vi "SetPara_BP4610.vi"(8 "error in":errorcluster, 10 "SetBP":T1={"Set"=enum."FREQ/WAVE", "Operation mode"=0, "Voltage[Vp-p]"=0.0, "Current[Ap-p]"=0.0, "Voltage[V]"=0.0, "Current[A]"=0.0, "Frequency[Hz]"=1.0, "Waveform"=enum."Sine"} {"Frequency[Hz]" min=1.0 max=100000.0 step=0.1; "Current[A]" min=-20.0 max=20.0 step=0.001; "Voltage[V]" min=-115.0 max=115.0 step=0.01; "Current[Ap-p]" min=0.0 max=60.0 step=0.01; "Voltage[Vp-p]" min=0.0 max=120.0 step=0.1; "Operation mode" items=["CV-INT", "CV-EXT", "CV-ADD", "CC-INT", "CC-EXT", "CC-ADD"]}, 11 "VISA":refnum<visa-resource-name> caption="VISAsession") -> (0 "error out":errorcluster, 3 "VISA out":refnum<visa-resource-name>)   [LabVIEW 2019]
uses:
  Type def/SetNF_BP4610.ctl
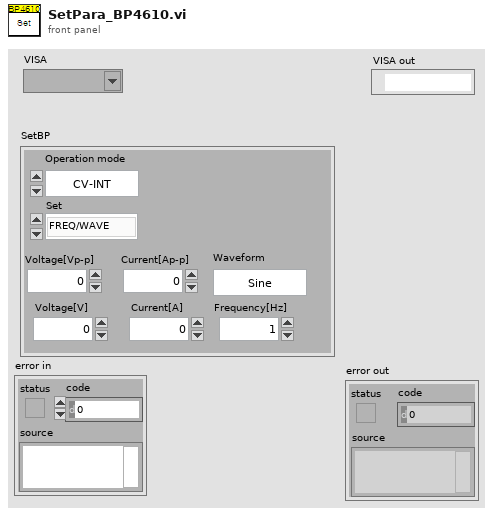
[diagram p1: front panel]
types:
  T1 = typedef "SetNF_BP4610.ctl" = cluster{"Set":enum16{"Current", "Voltage", "FREQ/WAVE"}, "Operation mode":u16, "Voltage[Vp-p]":dbl, "Current[Ap-p]":dbl, "Voltage[V]":dbl, "Current[A]":dbl, "Frequency[Hz]":dbl, "Waveform":enum16{"Sine", "Square", "ARB 1", "ARB 2", "ARB 3", "ARB 4", "ARB 5", "ARB 6", "ARB 7", "ARB 8", "ARB 9", "ARB 10", "ARB 11", "ARB 12", "ARB 13", "ARB 14", "ARB 15", "ARB 16"}}
  T2 = enum16{"Sine", "Square", "ARB 1", "ARB 2", "ARB 3", "ARB 4", "ARB 5", "ARB 6", "ARB 7", "ARB 8", "ARB 9", "ARB 10", "ARB 11", "ARB 12", "ARB 13", "ARB 14", "ARB 15", "ARB 16"}
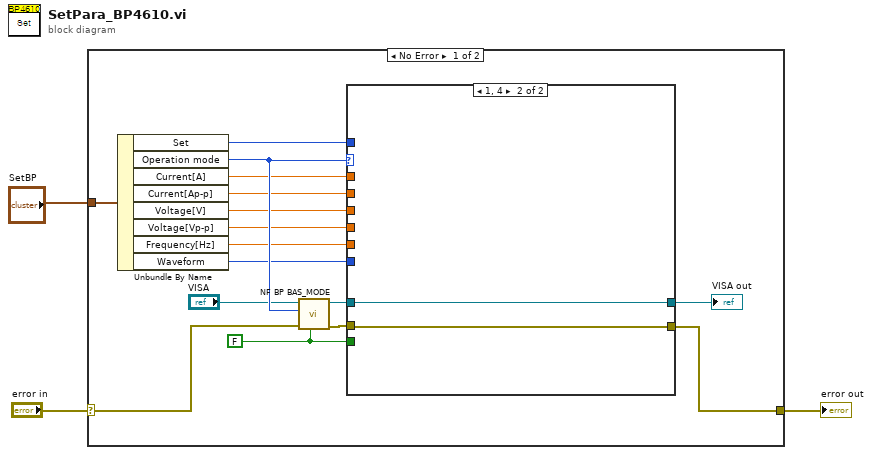
[diagram p0: block diagram]
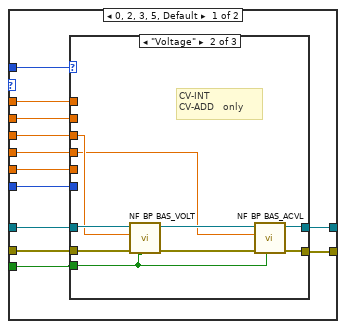
[diagram p2: hidden frame]
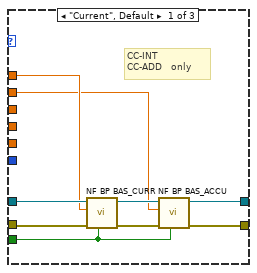
[diagram p3: hidden frame]
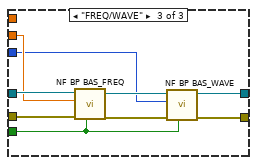
[diagram p4: hidden frame]
diagram:
  n1 = case shown="No Error" "error in" {
    selector: "error in" -> [w11 w61]
    tunnel: [w10 w61] -> w2
    tunnel: "SetBP" -> [w16 _]
    frame No Error {
      w17 = FALSE ("Read")
      n2 = Unbundle By Name(w16) -> ("Set"=w14:enum16{"Current", "Voltage", "FREQ/WAVE"}, "Operation mode"=w15:u16, "Current[A]"=w13:dbl, "Current[Ap-p]"=w12:dbl, "Voltage[V]"=w9:dbl, "Voltage[Vp-p]"=w8:dbl, "Frequency[Hz]"=w7:dbl, "Waveform"=w6:T2)
      n3 = call <instrlib>:"NF BP BAS_MODE.vi"("Read(F)"=w17, "error in (no error)"=w11, "Select Mode"=w15, "VISAsession"="VISA") -> ("error out"=w18:errorcluster, "CopyVISAsession"=w19:refnum<visa-resource-name>)  [unwired: 4 in, 2 out]
      n4 = case shown="1, 4" w15 {
        tunnel: w19 -> [w31 w60]
        tunnel: w18 -> [w30 w59]
        tunnel: [w29 w60] -> w4
        tunnel: [w28 w59] -> w10
        tunnel: w17 -> [w27 _]
        tunnel: w14 -> [w26 _]
        tunnel: w13 -> [w25 _]
        tunnel: w12 -> [w24 _]
        tunnel: w9 -> [w23 _]
        tunnel: w8 -> [w22 _]
        tunnel: w7 -> [w21 _]
        tunnel: w6 -> [w20 _]
        frame 0, 2, 3, 5, Default {
          n5 = case shown="\"Voltage\"" w26 {
            tunnel: w30 -> [w38 w49 w58]
            tunnel: w31 -> [w36 w45 w54]
            tunnel: [w40 w47 w55] -> w28
            tunnel: w27 -> [w37 w46 w56]
            tunnel: [w34 w43 w52] -> w29
            tunnel: w25 -> [w33 _ _]
            tunnel: w24 -> [w32 _ _]
            tunnel: w23 -> [_ w42 _]
            tunnel: w22 -> [_ w41 _]
            tunnel: w21 -> [_ _ w51]
            tunnel: w20 -> [_ _ w50]
            frame "Current", Default {
              # "CC-INT\nCC-ADD   only"
              n6 = call <instrlib>:"NF BP BAS_CURR.vi"("Read(F)"=w37, "error in (no error)"=w38, "Current[A]"=w33, "VISAsession"=w36) -> ("error out"=w39:errorcluster, "CopyVISAsession"=w35:refnum<visa-resource-name>)  [unwired: 4 in, 2 out]
              n7 = call <instrlib>:"NF BP BAS_ACCU.vi"("Read(F)"=w37, "error in (no error)"=w39, "Current[Ap-p]"=w32, "VISAsession"=w35) -> ("error out"=w40:errorcluster, "CopyVISAsession"=w34:refnum<visa-resource-name>)  [unwired: 4 in, 2 out]
            }
            frame "Voltage" {
              # "CV-INT\nCV-ADD   only"
              n8 = call <instrlib>:"NF BP BAS_VOLT.vi"("Read(F)"=w46, "error in (no error)"=w49, "Voltage[V]"=w42, "VISAsession"=w45) -> ("error out"=w48:errorcluster, "CopyVISAsession"=w44:refnum<visa-resource-name>)  [unwired: 4 in, 2 out]
              n9 = call <instrlib>:"NF BP BAS_ACVL.vi"("Read(F)"=w46, "error in (no error)"=w48, "Voltage[Vp-p]"=w41, "VISAsession"=w44) -> ("error out"=w47:errorcluster, "CopyVISAsession"=w43:refnum<visa-resource-name>)  [unwired: 4 in, 2 out]
            }
            frame "FREQ/WAVE" {
              n10 = call <instrlib>:"NF BP BAS_FREQ.vi"("Read(F)"=w56, "error in (no error)"=w58, "Frequency[Hz]"=w51, "VISAsession"=w54) -> ("error out"=w57:errorcluster, "CopyVISAsession"=w53:refnum<visa-resource-name>)  [unwired: 4 in, 2 out]
              n11 = call <instrlib>:"NF BP BAS_WAVE.vi"("Read(F)"=w56, "error in (no error)"=w57, "Select Function"=w50, "VISAsession"=w53) -> ("error out"=w55:errorcluster, "CopyVISAsession"=w52:refnum<visa-resource-name>)  [unwired: 4 in, 2 out]
            }
          }
        }
        frame 1, 4 {
        }
      }
      "VISA out" <- w4
    }
    frame Error {
    }
  }
  "error out" <- w2
